vi "Read_raw_inst_setup.vi"(0 "Setup file":string) -> (5 "Board type":T4=enum."Local ADAM", 6 "Local ADAM Channels":string[](array[string]), 8 "Setup string":string, 10 "Ch & spans choices":T5(array[cluster]) {"D" format="%.2f"; "Ch No" min=0; "low limit (-10V)" min=-10 max=10 format="%.2f"; "high limit (10V)" min=-10 max=10 format="%.2f"}, 13 "PWA Data":T1, 14 "Number of Analogue instruments":i32=1, 16 "LDA data":enum16{"No LDA data", "Take LDA data"}(ring)=enum."Take LDA data", 17 "LDA set up":T3={"dimensions"=enum."2D", "Arrival spacing"=FALSE, "Transit time"=FALSE}, 19 "Synchronise Analogue channels with LDA":bool)   [LabVIEW 2010]
uses:
  Controls/Inst_type.ctl
  Controls/Board_Types.ctl
  Controls/PWA_Data.ctl
  Controls/Post_Process.ctl
  File/Setup_Filetype.ctl
  Controls/Trigger_Mode.ctl
  Controls/Tunnel_Coordinates.ctl
  Globals/Meas_global.vi
  Globals/LDA_meas_global_1.vi
  Globals/LDA_meas_global_2.vi
  Globals/Trav_pos_global.vi
panel:
  in  "Inst type":T2
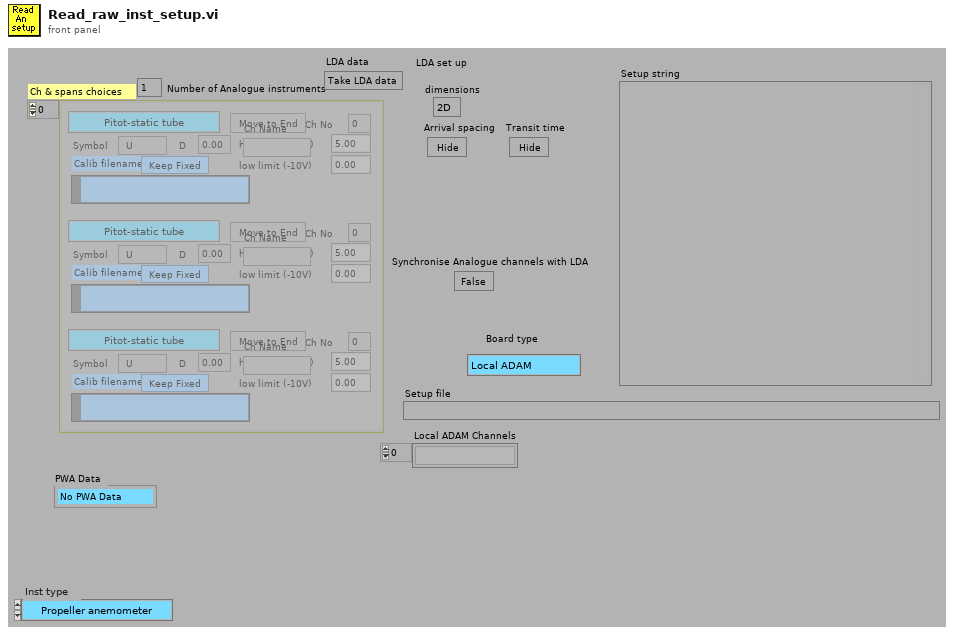
[diagram p1: front panel]
types:
  T1 = typedef "PWA_Data.ctl" = enum16{"No PWA Data", "One Ch PWA"}
  T2 = typedef "Inst_type.ctl" = enum16{"Propeller anemometer", "Raw voltage", "Pressure Transducer", "Pitot-static tube", "Preston tube", "Hot wire", "Cross wire 1", "Cross wire 2", "Generic Linear", "Generic Polynomial", "Generic BackPoly", "Fast FID", "Thermocouple", "Cold wire", "Pulsed Wire", "LDA Vel", "LDA Tran time", "LDA Arr time"}
  T3 = cluster{"dimensions":enum16{"1D", "2D"}, "Arrival spacing":bool, "Transit time":bool}
  T4 = typedef "Board_Types.ctl" = enum16{"Simulate", "Local ADAM", "Server ADAM", "NI-DAQmx", "NI-DAQmxBase", "ADC488", "DT LV-link"}
  T5 = cluster{"high limit (10V)":sgl, "low limit (-10V)":sgl, "Ch No":i16, "Calib filename":path, "Inst type":T2, "Symbol":string, "Move channel":bool, "Use Latest":bool, "D":dbl, "Ch Name":string}[]
  T6 = typedef "Post_Process.ctl" = enum16{"Take New Data", "Post Process Raw Data File"}
  T7 = typedef "Setup_Filetype.ctl" = enum16{"Measurement Setups", "Calibration Setups", "General", "Results File Plotter Setups", "Speed Calib Tweaks"}
  T8 = typedef "Trigger_Mode.ctl" = enum16{"Free Running", "Start on Trigger", "Trigger Every Block", "Trigger Every Sample"}
  T9 = typedef "Tunnel_Coordinates.ctl" = enum16{"Work in Tunnel Coordinates", "Work in Model Coordinates"}
  T10 = cluster{"high limit (10V)":sgl, "low limit (-10V)":sgl, "Ch No":i16, "Calib filename":path, "Inst type":T2, "Symbol":string, "Move channel":bool, "Use Latest":bool, "D":dbl, "Ch Name":string}
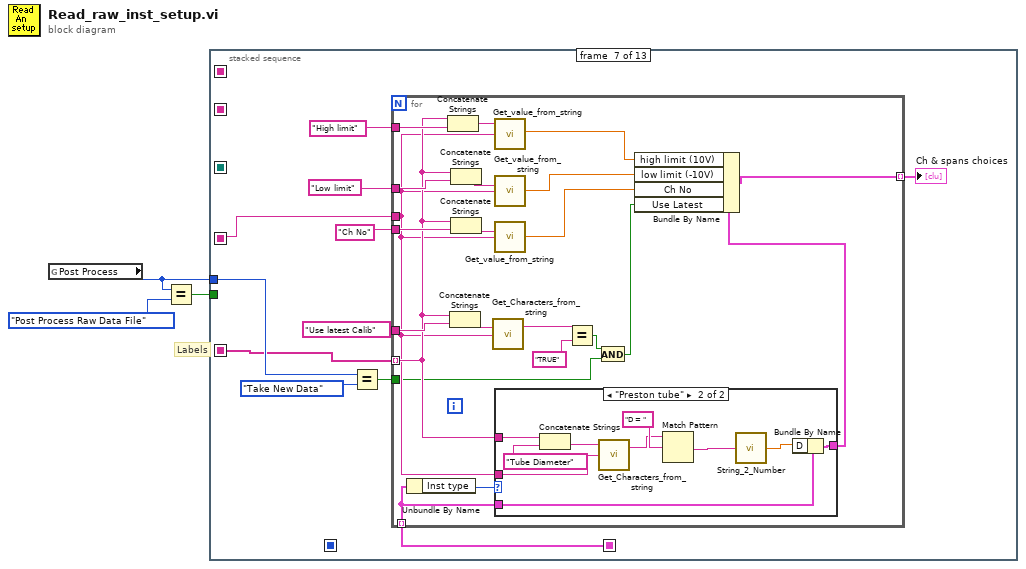
[diagram p0: block diagram]
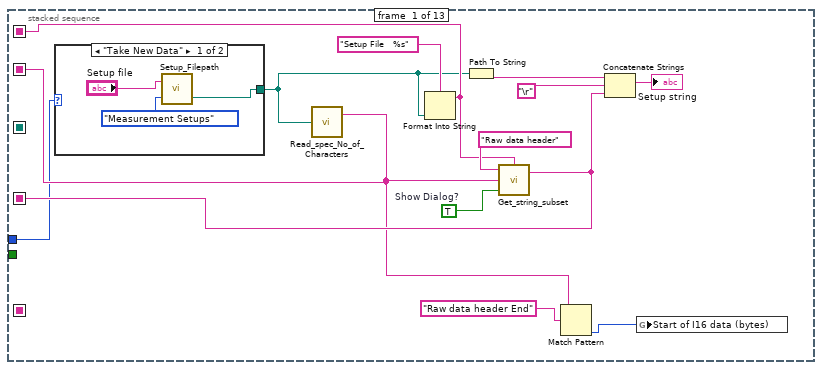
[diagram p2: hidden frame]
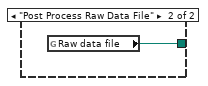
[diagram p3: hidden frame]
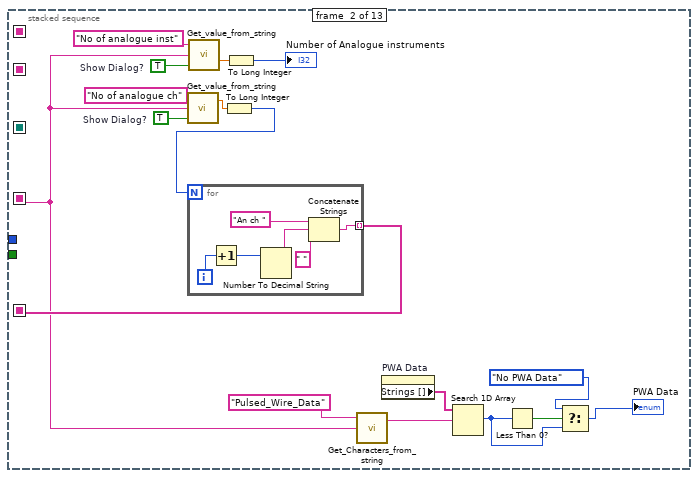
[diagram p4: hidden frame]
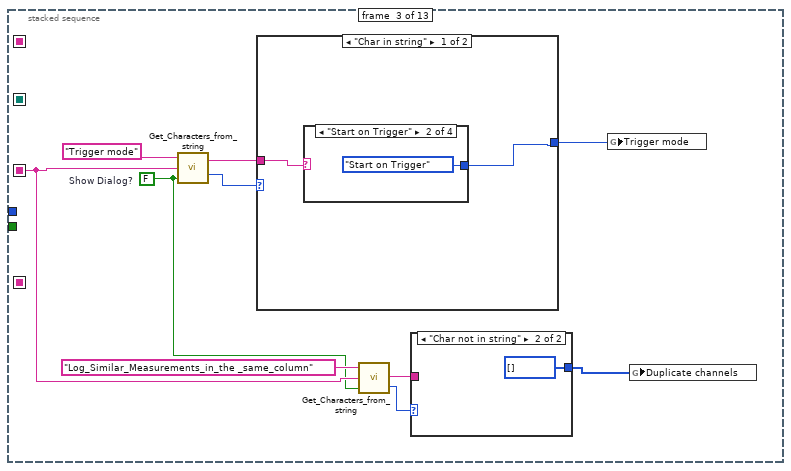
[diagram p5: hidden frame]
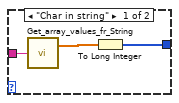
[diagram p6: hidden frame]
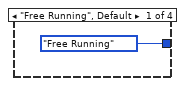
[diagram p7: hidden frame]
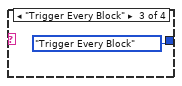
[diagram p8: hidden frame]
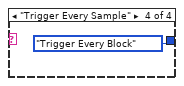
[diagram p9: hidden frame]
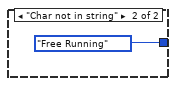
[diagram p10: hidden frame]
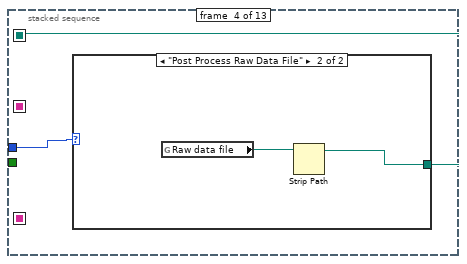
[diagram p11: hidden frame]
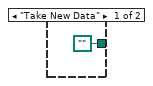
[diagram p12: hidden frame]
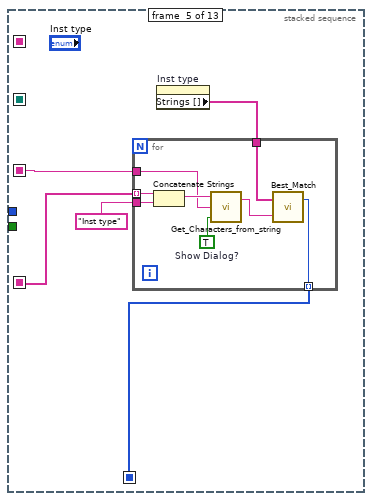
[diagram p13: hidden frame]
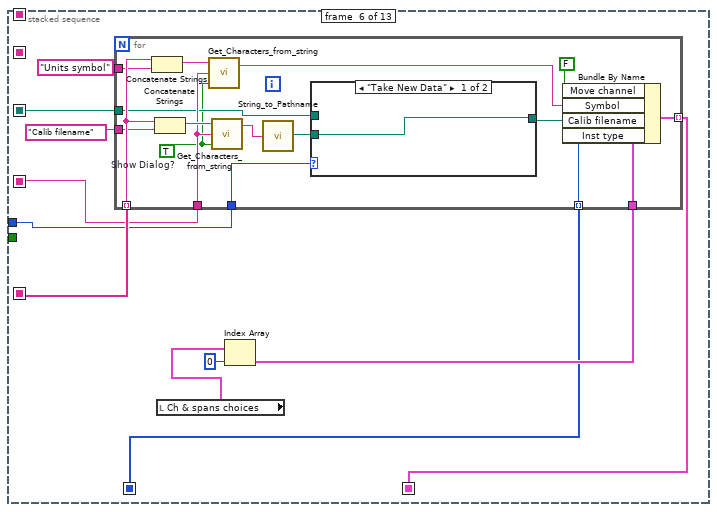
[diagram p14: hidden frame]
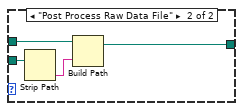
[diagram p15: hidden frame]
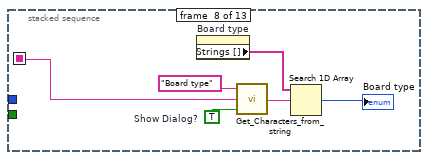
[diagram p17: hidden frame]
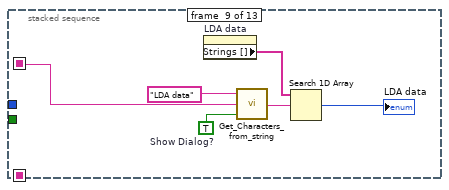
[diagram p18: hidden frame]
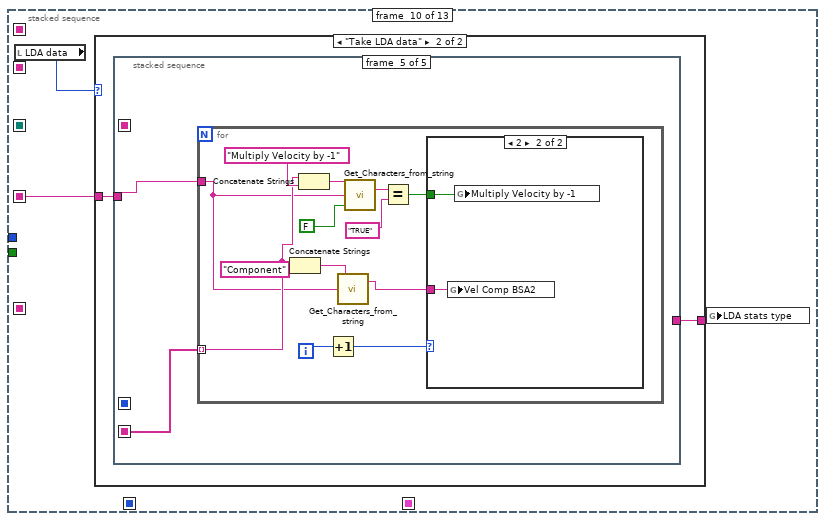
[diagram p19: hidden frame]
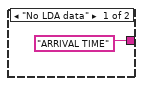
[diagram p20: hidden frame]
diagram:
  # "Labels"
  n1 = global read "Meas_global.vi" "Post Process"() -> (w1:T6)
  n2 = Equal?(x=w1, y=Post_Process."Post Process Raw Data File" ("Post Process")) -> (x = y?=w3:bool)
  n3 = stacked-sequence {
    seq-local: [w14 _ _ _ _ _ _ _ _ _ _ _ _] -> [_ w28 w48 _ w74 w84 w126 w164 w170 w174 w256 w283 w296]
    seq-local: [_ w35 _ _ _ _ _ _ _ _ _ _ _] -> [_ _ _ _ w73 w93 w117 _ _ _ _ _ _]
    seq-local: [_ _ _ _ w70 _ _ _ _ _ _ _ _] -> [_ _ _ _ _ w87 _ _ _ _ _ _ _]
    seq-local: [_ _ _ _ _ w86 _ _ _ _ _ _ _] -> [_ _ _ _ _ _ w125 _ _ _ _ _ _]
    seq-local: [_ _ _ w66 _ _ _ _ _ _ _ _ _] -> [_ _ _ _ _ w85 _ _ _ _ _ _ _]
    seq-local: [w9 _ _ _ _ _ _ _ _ _ _ _ _] -> [_ _ _ _ _ _ _ _ _ _ _ _ w295]
    seq-local: [w6 _ _ _ _ _ _ _ _ _ _ _ _] -> [_ _ _ _ _ _ _ _ _ _ _ w279 _]
    tunnel: w3 -> [_ _ _ _ _ _ _ _ _ _ _ _ w297]
    tunnel: w1 -> [w5 _ _ w65 _ w83 w118 _ _ _ _ w280 _]
    frame #0 {
      w11 = TRUE  # Show Dialog?
      n4 = case shown="\"Take New Data\"" w5 {
        tunnel: [w17 w20] -> w4
        frame "Take New Data" {
          n5 = call "Setup_Filepath.vi"("Setup File Type"=Setup_Filetype."Measurement Setups", "Filename in"="Setup file") -> ("Filename Out"=w17:path)  [unwired: 1 out]
        }
        frame "Post Process Raw Data File" {
          n6 = global read "Meas_global.vi" "Raw data file"() -> (w20:path)
        }
      }
      n7 = call "Read_spec_No_of_Characters.vi"("Filename"=w4) -> ("character string"=w9:string)  [unwired: 1 out]
      n8 = Format Into String(format string="Setup File   %s", w4) -> (resulting string=w6:string)  [unwired: 2 in, 1 out]
      n9 = Path To String(path=w4) -> (string=w12:string)
      n10 = call "Get_string_subset.vi"("String Name"=w6, "Show Dialog?"=w11, "String to split"=w9, "File Label"="Raw data header") -> ("Output string"=w14:string)  [unwired: 1 out]
      n11 = Match Pattern(string=w9, regular expression="Raw data header End") -> (offset past match=w8:i32)  [unwired: 4 out]
      n12 = Concatenate Strings(w12, "\r", w14) -> (→"Setup string":string)
      n13 = global write "Meas_global.vi" "Start of I16 data (bytes)"(w8) -> ()
    }
    frame #1 {
      w29 = TRUE  # Show Dialog?
      w30 = TRUE  # Show Dialog?
      n14 = call "Get_value_from_string.vi"("Show Dialog?"=w30, "Input string"=w28, "Variable name"="No of analogue ch") -> ("Value"=w36:dbl)  [unwired: 1 out]
      n15 = call "Get_value_from_string.vi"("Show Dialog?"=w29, "Input string"=w28, "Variable name"="No of analogue inst") -> ("Value"=w33:dbl)  [unwired: 1 out]
      n16 = To Long Integer(number=w36) -> (32bit integer=w31:i32)
      n17 = for {
        N: w31 -> [_]
        tunnel: [w39] -> w35 mode=indexing
        i -> [w41]
        n18 = Increment(x=w41) -> (x+1=w40:i32)
        n19 = Number To Decimal String(number=w40) -> (decimal integer string=w43:string)  [unwired: 1 out]
        n20 = Concatenate Strings("An ch ", w43, " ") -> (w39:string)
      }
      n21 = To Long Integer(number=w33) -> (32bit integer=→"Number of Analogue instruments":i32)
      n22 = call "Get_Characters_from_string.vi"("Input string"=w28, "Variable name"="Pulsed_Wire_Data") -> ("Value"=w25:string)  [unwired: 1 in, 1 out]
      n23 = property on="PWA Data" class="Enum (strict)"() -> ("Strings []"=w26:string[])  [unwired: 2 in, 2 out]
      n24 = Search 1D Array(1D array=w26, element=w25) -> (index of element=w22:i32)  [unwired: 1 out]
      n25 = Less Than 0?(x=w22) -> (x < 0?=w24:bool)
      n26 = Select(t=PWA_Data."No PWA Data" ("PWA Data"), s=w24, f=w22) -> (s? t:f=→"PWA Data":i32)
    }
    frame #2 {
      w47 = FALSE  # Show Dialog?
      n27 = call "Get_Characters_from_string.vi"("Show Dialog?"=w47, "Input string"=w48, "Variable name"="Trigger mode") -> ("Status"=w52:enum16{"Char in string", "Char not in string"}, "Value"=w51:string)
      n28 = case shown="\"Char in string\"" w52 {
        tunnel: [w58 Trigger_Mode."Free Running" ("Trigger mode")] -> w50
        tunnel: w51 -> [w59 _]
        frame "Char in string" {
          n29 = case shown="\"Start on Trigger\"" w59 {
            tunnel: [Trigger_Mode."Free Running" ("Trigger mode") Trigger_Mode."Start on Trigger" ("Trigger mode") Trigger_Mode."Trigger Every Block" ("Trigger mode") Trigger_Mode."Trigger Every Block" ("Trigger mode")] -> w58
            frame "Free Running", Default {
            }
            frame "Start on Trigger" {
            }
            frame "Trigger Every Block" {
            }
            frame "Trigger Every Sample" {
            }
          }
        }
        frame "Char not in string" {
        }
      }
      n30 = call "Get_Characters_from_string.vi"("Show Dialog?"=w47, "Input string"=w48, "Variable name"="Log_Similar_Measurements_in_the _same_column") -> ("Status"=w44:enum16{"Char in string", "Char not in string"}, "Value"=w46:string)
      n31 = case shown="\"Char not in string\"" w44 {
        tunnel: w46 -> [w56 _]
        tunnel: [w54 i32[] []] -> w45
        frame "Char in string" {
          n32 = call "Get_array_values_fr_String.vi"("String Value"=w56) -> ("Numeric Array"=w55:dbl[])  [unwired: 1 out]
          n33 = To Long Integer(number=w55) -> (32bit integer=w54:i32[])
        }
        frame "Char not in string" {
        }
      }
      n34 = global write "Meas_global.vi" "Trigger mode"(w50) -> ()
      n35 = global write "Meas_global.vi" "Duplicate channels"(w45) -> ()
    }
    frame #3 {
      n36 = case shown="\"Post Process Raw Data File\"" w65 {
        tunnel: [path "" ("stripped path") w68] -> w66
        frame "Take New Data" {
        }
        frame "Post Process Raw Data File" {
          n37 = global read "Meas_global.vi" "Raw data file"() -> (w69:path)
          n38 = Strip Path(path=w69) -> (stripped path=w68:path)  [unwired: 1 out]
        }
      }
    }
    frame #4 {
      n39 = property on="Inst type" class="Enum (strict)"() -> ("Strings []"=w71:string[])  [unwired: 2 in, 2 out]
      n40 = for {
        tunnel: w74 -> [w81]
        tunnel: w71 -> [w77]
        tunnel: w73 -> [w80] mode=indexing
        tunnel: "Inst type" -> [w79]
        tunnel: [w75] -> w70 mode=indexing
        w78 = TRUE  # Show Dialog?
        n41 = Concatenate Strings(w80, w79) -> (w82:string)
        n42 = call "Get_Characters_from_string.vi"("Show Dialog?"=w78, "Input string"=w81, "Variable name"=w82) -> ("Value"=w76:string)  [unwired: 1 out]
        n43 = call "Best_Match.vi"("Input String"=w76, "String Options"=w77) -> ("index of element"=w75:i32)  [unwired: 1 out]
      }
    }
    frame #5 {
      n44 = local read "Ch & spans choices"() -> (w89:T5)
      n45 = Index Array(array=w89, index=0) -> (element=w88:T10)
      n46 = for {
        tunnel: w93 -> [w108] mode=indexing
        tunnel: "Calib filename" -> [w107]
        tunnel: "Units symbol" -> [w106]
        tunnel: w88 -> [w105]
        tunnel: w87 -> [w103] mode=indexing
        tunnel: [w102] -> w86 mode=indexing
        tunnel: w84 -> [w101]
        tunnel: w83 -> [w100]
        tunnel: w85 -> [w99]
        w96 = TRUE  # Show Dialog?
        n47 = Concatenate Strings(w108, w106) -> (w110:string)
        n48 = Concatenate Strings(w108, w107) -> (w109:string)
        n49 = call "Get_Characters_from_string.vi"("Show Dialog?"=w96, "Input string"=w101, "Variable name"=w110) -> ("Value"=w104:string)  [unwired: 1 out]
        n50 = call "Get_Characters_from_string.vi"("Show Dialog?"=w96, "Input string"=w101, "Variable name"=w109) -> ("Value"=w95:string)  [unwired: 1 out]
        n51 = call "String_to_Pathname.vi"("Input String"=w95) -> ("path"=w94:path)
        n52 = case shown="\"Take New Data\"" w100 {
          tunnel: w94 -> [w111 w115]
          tunnel: w99 -> [_ w112]
          tunnel: [w111 w113] -> w98
          frame "Take New Data" {
          }
          frame "Post Process Raw Data File" {
            n53 = Strip Path(path=w115) -> (name=w114:string)  [unwired: 1 out]
            n54 = Build Path(base path=w112, name or relative path=w114) -> (appended path=w113:path)
          }
        }
        n55 = Bundle By Name(cluster=w105, "Move channel"=FALSE, "Symbol"=w104, "Calib filename"=w98, "Inst type"=w103) -> (w102:T10)
      }
    }
    frame #6 {
      n56 = Equal?(x=w118, y=Post_Process."Take New Data" ("Post Process")) -> (x = y?=w116:bool)
      n57 = for {
        tunnel: "Low limit" -> [w148]
        tunnel: "High limit" -> [w147]
        tunnel: w125 -> [w129] mode=indexing
        tunnel: [w139] -> w124 mode=indexing
        tunnel: w126 -> [w131]
        tunnel: "Ch No" -> [w143]
        tunnel: "Use latest Calib" -> [w137]
        tunnel: w117 -> [w132] mode=indexing
        tunnel: w116 -> [w130]
        n58 = Unbundle By Name(w129) -> ("Inst type"=w133:T2)
        n59 = Concatenate Strings(w132, w147) -> (w146:string)
        n60 = Concatenate Strings(w132, w137) -> (w138:string)
        n61 = Concatenate Strings(w132, w148) -> (w145:string)
        n62 = Concatenate Strings(w132, w143) -> (w144:string)
        n63 = call "Get_Characters_from_string.vi"("Input string"=w131, "Variable name"=w138) -> ("Value"=w136:string)  [unwired: 1 in, 1 out]
        n64 = call "Get_value_from_string.vi"("Input string"=w131, "Variable name"=w146) -> ("Value"=w142:dbl)  [unwired: 1 in, 1 out]
        n65 = call "Get_value_from_string.vi"("Input string"=w131, "Variable name"=w145) -> ("Value"=w141:dbl)  [unwired: 1 in, 1 out]
        n66 = call "Get_value_from_string.vi"("Input string"=w131, "Variable name"=w144) -> ("Value"=w140:dbl)  [unwired: 1 in, 1 out]
        n67 = case shown="\"Preston tube\"" w133 {
          tunnel: w132 -> [_ w159]
          tunnel: w131 -> [_ w154]
          tunnel: w129 -> [w149 w157]
          tunnel: [w149 w156] -> w128
          frame "Propeller anemometer", Default {
          }
          frame "Preston tube" {
            n68 = Concatenate Strings(w159, "Tube Diameter") -> (w155:string)
            n69 = call "Get_Characters_from_string.vi"("Input string"=w154, "Variable name"=w155) -> ("Value"=w152:string)  [unwired: 1 in, 1 out]
            n70 = Match Pattern(string=w152, regular expression="D = " ("String to match")) -> (after substring=w151:string)  [unwired: 4 out]
            n71 = call "String_2_Number.vi"("Value"=w151) -> ("Numeric"=w150:dbl)
            n72 = Bundle By Name(cluster=w157, "D"=w150) -> (w156:T10)
          }
        }
        n73 = Equal?(x=w136, y="TRUE") -> (x = y?=w134:bool)
        n74 = And(x=w134, y=w130) -> (x .and. y?=w127:bool)
        n75 = Bundle By Name(cluster=w128, "high limit (10V)"=w142, "low limit (-10V)"=w141, "Ch No"=w140, "Use Latest"=w127) -> (w139:T10)
      }
      "Ch & spans choices" <- w124
    }
    frame #7 {
      w161 = TRUE  # Show Dialog?
      n76 = property on="Board type" class="Enum (strict)"() -> ("Strings []"=w160:string[])  [unwired: 2 in, 2 out]
      n77 = call "Get_Characters_from_string.vi"("Show Dialog?"=w161, "Input string"=w164, "Variable name"="Board type") -> ("Value"=w165:string)  [unwired: 1 out]
      n78 = Search 1D Array(1D array=w160, element=w165) -> (index of element=→"Board type":i32)  [unwired: 1 out]
    }
    frame #8 {
      w167 = TRUE  # Show Dialog?
      n79 = property on="LDA data" class="Enum (strict)"() -> ("Strings []"=w166:string[])  [unwired: 2 in, 2 out]
      n80 = call "Get_Characters_from_string.vi"("Show Dialog?"=w167, "Input string"=w170, "Variable name"="LDA data" ("Label for characters")) -> ("Value"=w171:string)  [unwired: 1 out]
      n81 = Search 1D Array(1D array=w166, element=w171) -> (index of element=→"LDA data":i32)  [unwired: 1 out]
    }
    frame #9 {
      n82 = local read "LDA data"() -> (w173:enum16{"No LDA data", "Take LDA data"})
      n83 = case shown="\"Take LDA data\"" w173 {
        tunnel: w174 -> [_ w177]
        tunnel: ["ARRIVAL TIME" ("Adam client setup name") w176] -> w172
        frame "No LDA data" {
        }
        frame "Take LDA data" {
          n84 = stacked-sequence {
            seq-local: [_ w183 _ _ _] -> [_ _ _ w227 _]
            seq-local: [_ _ _ w226 _] -> [_ _ _ _ w237]
            seq-local: [w178 _ _ _ _] -> [_ w186 _ _ _]
            tunnel: w177 -> [_ w182 w216 _ w238]
            tunnel: [_ _ w215 _ _] -> w176
            frame #0 {
              n85 = Build Array("LDA Transit Time", "LDA Arrival spacing", "LDA Dimensions") -> (w178:string[])
            }
            frame #1 {
              n86 = local read "LDA set up"() -> (w185:T3)
              n87 = for {
                tunnel: w186 -> [w192] mode=indexing
                shift-right: [w189] -> w184
                shift-left: w185 -> [w190]
                tunnel: w182 -> [w187]
                n88 = call "Get_Characters_from_string.vi"("Input string"=w187, "Variable name"=w192) -> ("Status"=w191:enum16{"Char in string", "Char not in string"}, "Value"=w188:string)  [unwired: 1 in]
                n89 = case shown="\"Char in string\"" w191 {
                  tunnel: w192 -> [w196 _]
                  tunnel: w190 -> [w195 w214]
                  tunnel: [w194 w214] -> w189
                  tunnel: w188 -> [w193 _]
                  frame "Char in string" {
                    n90 = case shown="\"LDA Arrival spacing\"" w196 {
                      tunnel: w195 -> [w200 w203 w208 w213]
                      tunnel: [w199 w203 w207 w212] -> w194
                      tunnel: w193 -> [w198 _ w206 w211]
                      frame "LDA Dimensions" {
                        n91 = case shown="\"2D\", Default" w198 {
                          tunnel: [enum16{"1D", "2D"}."1D" ("Bundle Element") enum16{"1D", "2D"}."2D" ("Bundle Element")] -> w197
                          frame "1D" {
                          }
                          frame "2D", Default {
                          }
                        }
                        n92 = Bundle By Name(cluster=w200, "dimensions"=w197) -> (w199:T3)
                      }
                      frame "No Match", Default {
                      }
                      frame "LDA Arrival spacing" {
                        n93 = Equal?(x=w206, y="TRUE") -> (x = y?=w204:bool)
                        n94 = Bundle By Name(cluster=w208, "Arrival spacing"=w204) -> (w207:T3)
                      }
                      frame "LDA Transit Time" {
                        n95 = Equal?(x=w211, y="TRUE") -> (x = y?=w209:bool)
                        n96 = Bundle By Name(cluster=w213, "Transit time"=w209) -> (w212:T3)
                      }
                    }
                  }
                  frame "Char not in string" {
                  }
                }
              }
              "LDA set up" <- w184
              n97 = Unbundle By Name(w184) -> ("dimensions"=w183:enum16{"1D", "2D"})
            }
            frame #2 {
              n98 = call "Get_Characters_from_string.vi"("Input string"=w216, "Variable name"="LDA stats weighting") -> ("Status"=w219:enum16{"Char in string", "Char not in string"}, "Value"=w218:string)  [unwired: 1 in]
              n99 = case shown="\"Char in string\"" w219 {
                tunnel: "ARRIVAL TIME" ("Adam client setup name") -> [w223 w225]
                tunnel: w218 -> [w222 _]
                tunnel: [w221 w225] -> w215
                frame "Char in string" {
                  n100 = Empty String/Path?(string/path=w222) -> (empty?=w224:bool)
                  n101 = Select(t=w223, s=w224, f=w222) -> (s? t:f=w221:string)
                }
                frame "Char not in string" {
                }
              }
            }
            frame #3 {
              n102 = case shown="\"1D\"" w227 {
                tunnel: [1 2] -> w228
                frame "1D" {
                }
                frame "2D" {
                }
              }
              n103 = for {
                N: w228 -> [_]
                tunnel: [w230] -> w226 mode=indexing
                i -> [w232]
                n104 = Increment(x=w232) -> (x+1=w231:i32)
                n105 = Number To Decimal String(number=w231) -> (decimal integer string=w234:string)  [unwired: 1 out]
                n106 = Concatenate Strings("BSA ", w234, " ") -> (w230:string)
              }
            }
            frame #4 {
              n107 = for {
                tunnel: w238 -> [w240]
                tunnel: w237 -> [w241] mode=indexing
                i -> [w250]
                n108 = Concatenate Strings(w241, "Component") -> (w251:string)
                n109 = Concatenate Strings(w241, "Multiply Velocity by -1") -> (w245:string)
                n110 = Increment(x=w250) -> (x+1=w247:i32)
                n111 = call "Get_Characters_from_string.vi"("Input string"=w240, "Variable name"=w251) -> ("Value"=w248:string)  [unwired: 1 in, 1 out]
                n112 = call "Get_Characters_from_string.vi"("Show Dialog?"=FALSE, "Input string"=w240, "Variable name"=w245) -> ("Value"=w243:string)  [unwired: 1 out]
                n113 = Equal?(x=w243, y="TRUE") -> (x = y?=w239:bool)
                n114 = case shown="2" w247 {
                  tunnel: w248 -> [w253 w255]
                  tunnel: w239 -> [w252 w254]
                  frame 1, Default {
                    n115 = global write "LDA_meas_global_1.vi" "Vel Comp BSA1"(w253) -> ()
                    n116 = global write "LDA_meas_global_1.vi" "Multiply Velocity by -1"(w252) -> ()
                  }
                  frame 2 {
                    n117 = global write "LDA_meas_global_2.vi" "Vel Comp BSA2"(w255) -> ()
                    n118 = global write "LDA_meas_global_2.vi" "Multiply Velocity by -1"(w254) -> ()
                  }
                }
              }
            }
          }
        }
      }
      n119 = global write "LDA_meas_global_1.vi" "LDA stats type"(w172) -> ()
    }
    frame #10 {
      n120 = Build Array("Synchronise with LDA") -> (w266:string[])
      n121 = Build Array("FALSE", "TRUE") -> (w263:string[])
      n122 = call "Get_value_from_string.vi"("Input string"=w256, "Variable name"="Sync Delay Time (ms)" ("Label for characters")) -> ("Status"=w258:enum16{"Char in string", "Char not in string"}, "Value"=w257:dbl)  [unwired: 1 in]
      n123 = case shown="\"Char in string\"" w258 {
        tunnel: w257 -> [w268 _]
        frame "Char in string" {
          n124 = global write "LDA_meas_global_1.vi" "Sync Delay Time (ms)"(w268) -> ()
        }
        frame "Char not in string" {
        }
      }
      n125 = Build Array(FALSE, TRUE) -> (w260:bool[])
      n126 = for {
        tunnel: w256 -> [w276]
        tunnel: w266 -> [w272] mode=indexing
        tunnel: w263 -> [w271]
        tunnel: w260 -> [w270]
        i -> [w274]
        w269 = TRUE  # Show Dialog?
        n127 = call "Get_Characters_from_string.vi"("Show Dialog?"=w269, "Input string"=w276, "Variable name"=w272) -> ("Value"=w277:string)  [unwired: 1 out]
        n128 = Search 1D Array(1D array=w271, element=w277) -> (index of element=w275:i32)  [unwired: 1 out]
        n129 = Index Array(array=w270, index=w275) -> (element=w273:bool)
        n130 = case shown="1" w274 {
          tunnel: w273 -> [w278 _]
          frame 0, Default {
            "Synchronise Analogue channels with LDA" <- w278
          }
          frame 1 {
          }
        }
      }
    }
    frame #11 {
      n131 = Build Array("Local ADAM Channels") -> (w282:string[])
      n132 = for {
        tunnel: w283 -> [w289]
        tunnel: w282 -> [w288] mode=indexing
        tunnel: w280 -> [w285]
        tunnel: w279 -> [w284]
        i -> [w287]
        n133 = call "Get_string_subset.vi"("String Name"=w284, "String to split"=w289, "File Label"=w288) -> ("Output string"=w293:string)  [unwired: 1 in, 1 out]
        n134 = Initialize Array("") -> (w286:string[])  [unwired: 1 out]
        n135 = Spreadsheet String To Array(format string="%s", spreadsheet string=w293, array type (2D Dbl)=w286) -> (array=w290:string[])  [unwired: 1 out]
        n136 = case shown="0, Default" w287 {
          tunnel: w290 -> [w294]
          tunnel: w285 -> [_]
          frame 0, Default {
            "Local ADAM Channels" <- w294
          }
        }
      }
    }
    frame #12 {
      n137 = case shown="True" w297 {
        tunnel: w296 -> [_ w303]
        tunnel: w295 -> [_ w298]
        frame False {
        }
        frame True {
          w302 = FALSE  # Show Dialog?
          n138 = call "Get_Characters_from_string.vi"("Show Dialog?"=w302, "Input string"=w303, "Variable name"="Coordinate_System" ("Label for characters")) -> ("Status"=w301:enum16{"Char in string", "Char not in string"}, "Value"=w300:string)
          n139 = case shown="\"Char not in string\"" w301 {
            tunnel: w300 -> [w306 _]
            tunnel: [w305 w309] -> w299
            tunnel: w298 -> [_ w311]
            frame "Char in string" {
              n140 = case shown="\"Work in Model Coordinates\"" w306 {
                tunnel: [Tunnel_Coordinates."Work in Model Coordinates" ("Work in Tunnel Coordinates?") Tunnel_Coordinates."Work in Tunnel Coordinates" ("Work in Tunnel Coordinates?")] -> w305
                frame "Work in Model Coordinates" {
                }
                frame "Work in Tunnel Coordinates", Default {
                }
              }
            }
            frame "Char not in string" {
              n141 = Concatenate Strings("X Pos (Model)", "\t", "Y Pos (Model)") -> (w312:string)
              n142 = Match Pattern(string=w311, regular expression=w312) -> (offset past match=w310:i32)  [unwired: 4 out]
              n143 = case shown="-1" w310 {
                tunnel: [Tunnel_Coordinates."Work in Model Coordinates" ("Work in Tunnel Coordinates?") Tunnel_Coordinates."Work in Tunnel Coordinates" ("Work in Tunnel Coordinates?")] -> w309
                frame 0, Default {
                }
                frame -1 {
                }
              }
            }
          }
          n144 = global write "Trav_pos_global.vi" "Work in Tunnel Coordinates?"(w299) -> ()
        }
      }
    }
  }
